vi "ATE_Bandwidth.vi"() -> ()   [LabVIEW 2009]
doc: "Use this template to build a producer/consumer design pattern with events to produce queue items. Use this design pattern instead of the User Interface Event Handler pattern for user interfaces when you want to execute code asynchronously in response to an event without slowing the user interface responsiveness."
uses:
  Rvp8PowerData.ctl
  <vilib>/Analysis/NI_AALPro.lvlib
panel:
  in  "Ready":bool
  out "Instructions":string="rvp8 bandwidth measuring vi\n\nBasic operation:\u0000\u0000\n1 - configure ATE switches with the yellow 'Bandwidth Setup' button\u0000\u0000\n2 - measure the bandwidth with the red 'Calibrate' button\n3 - exit the program with the red 'Exit' button\n\nHints:\nWait for the green 'READY' light before clicking buttons\nClick appropriate blue buttons after making changes on 'Controls' tab\nCheck status tab before calibration"
  out "Real Time XY":cluster{dbl[], dbl[]}(graph)
  in  "Configuration 1":bool
  out "Cal Output File":path
  out "?":cluster{dbl[], dbl[]}[](graph)
  out "RVP8 Bandwidth":cluster{dbl[], dbl[]}[](graph)
  in  "DataSource":bool
  out "File Name":string
  in  "Data Directory":string="/home/operator/ate/data/rvp8_bw"
  in  "Set SigGen":bool
  in  "Initialize":bool
  in  "70 dB":bool
  in  "121 dB":bool
  in  "Switches":bool
  in  "Calibrate":bool
  in  "Stop":bool
  in  "ATE TABS":enum32{"Status", "Controls"}(tab)=enum."Controls"
  out "ATE Switch Status":T1
  out "121dB\nAttenuators":bool[](array[boolean])
  out "70dB\nAttenuators":bool[](array[boolean])
  out "RVP8 Power":T2 {"time" format="%<%H:%M:%S\n%Y/%m/%d>T"}
  out "Signal Generator Status":T3={"Freq (GHz)"=0.0, "RF Power (dBm)"=0.0, "RF Power"=TRUE} {"Freq (GHz)" format="%.5g"; "RF Power (dBm)" format="%.2g"}
  out "121 Verified":bool
  out "70 Verfied":bool
  in  "Center Frequency (GHz)":dbl=2.809 format="%.5g"
  in  "Steps":i32=51
  in  "Steps Size (GHz)":dbl=0.0001 min=0.0 max=0.002 step=1e-06 format="%.5g"
  in  "70 dB Attn":i32=70 min=0 max=70 step=10
  in  "121 dB Attn":i32=121 min=0 max=121 step=1
  in  "ATE Switches":T4
  out "P-State":string
  out "C-State":string
  in  "Busy":bool
  # "RVP8 Bandwidth"
  # "1 dB"
  # "2 dB"
  # "4 dB"
  # "4 dB"
  # "10 dB"
  # "20 dB"
  # "40 dB"
  # "40 dB"
  # "10 dB"
  # "20 dB"
  # "40 dB"
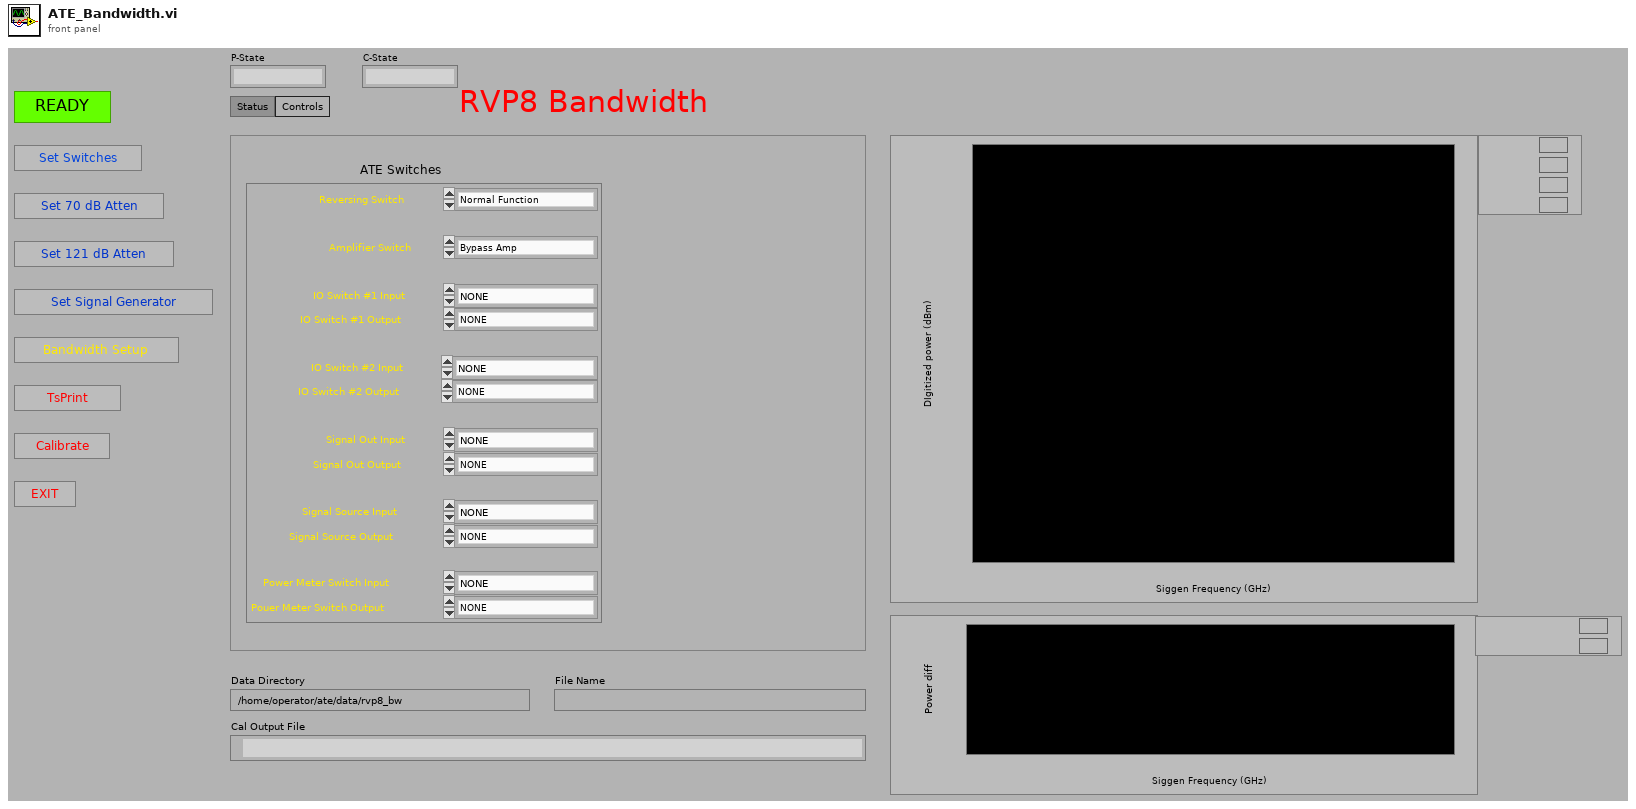
[diagram p1: front panel]
types:
  T1 = cluster{"Reversing Switch ":bool, "IO Switch #1":bool, "IO Switch #2":bool, "Signal Out":bool, "Signal Source":bool, "Power Meter":bool, "Amp By Pass":bool}
  T2 = typedef "Rvp8PowerData.ctl" = cluster{"success":bool, "time":dbl, "el":dbl, "az":dbl, "dbm0":dbl, "dbm1":dbl, "dbmHc":dbl, "dbmHx":dbl, "dbmVc":dbl, "dbmVx":dbl}
  T3 = cluster{"Freq (GHz)":dbl, "RF Power (dBm)":dbl, "RF Power":bool}
  T4 = cluster{"Reversing Switch":enum16{"Normal Function", "Reversing Function"}, "IO Switch #1 Input":enum16{"NONE", "AHR (J2)", "Splitter", "Signal Out Switch (S3)", "Reversing Switch"}, "IO Switch #1 Output":enum16{"NONE", "AHR (J2)", "Delay Device (S4)", "Power Meter Switch (S5)", "Reversing Switch"}, "IO Switch #2 Input":enum16{"NONE", "AVR (J3)", "Splitter", "Signal Out Switch (S3)", " 2W Term (TM1)", "Reversing Switch"}, "IO Switch #2 Output":enum16{"NONE", "AVR (J3)", "Signal Out Switch (S3)", "Power Meter Switch (S5)", "Reversing Switch", "2W Term (TM1)"}, "Signal Out Input":enum16{"NONE", "Amp Bypass Switch (S6)", "IO Switch #1 (S1)", "IO Switch #2 (S2)", "2W Term (TM3)"}, "Signal Out Output":enum16{"NONE", "2 Watt Term (TM3)", "Splitter", "Power Meter Switch (S5)"}, "Signal Source Input":enum16{"NONE", "Delay Device", "Signal Generator (J7)", "Inside Noise Box NF (J5)", "2W Term (TM3)"}, "Signal Source Output":enum16{"NONE", "Amp Bypass Switch", "Test Pulse Generator", "Power Meter Switch (S5)"}, "Power Meter Switch Input":enum16{"NONE", "IO Switch #1 (S1)", "Signal Source Switch (S4)", "Signal Out Switch (S3)", "IO Switch #2 (S2)", "TXH-TXV Switch (J8)"}, "Pouer Meter Switch Output":enum16{"NONE", "Power Meter (J6)"}, "Amplifier Switch":enum16{"Bypass Amp", "Include Amp"}}
  T5 = cluster{"Frequency (GHz)":dbl, "RF Power (dBm)":dbl, "RF ON/OFF":bool}
  T6 = enum16{"open", "replace", "create", "open or create", "replace or create", "replace or create with confirmation"}
  T7 = cluster{"Frequency (GHz)":dbl, "RF Power (dBm)":dbl, "RF Power":bool}
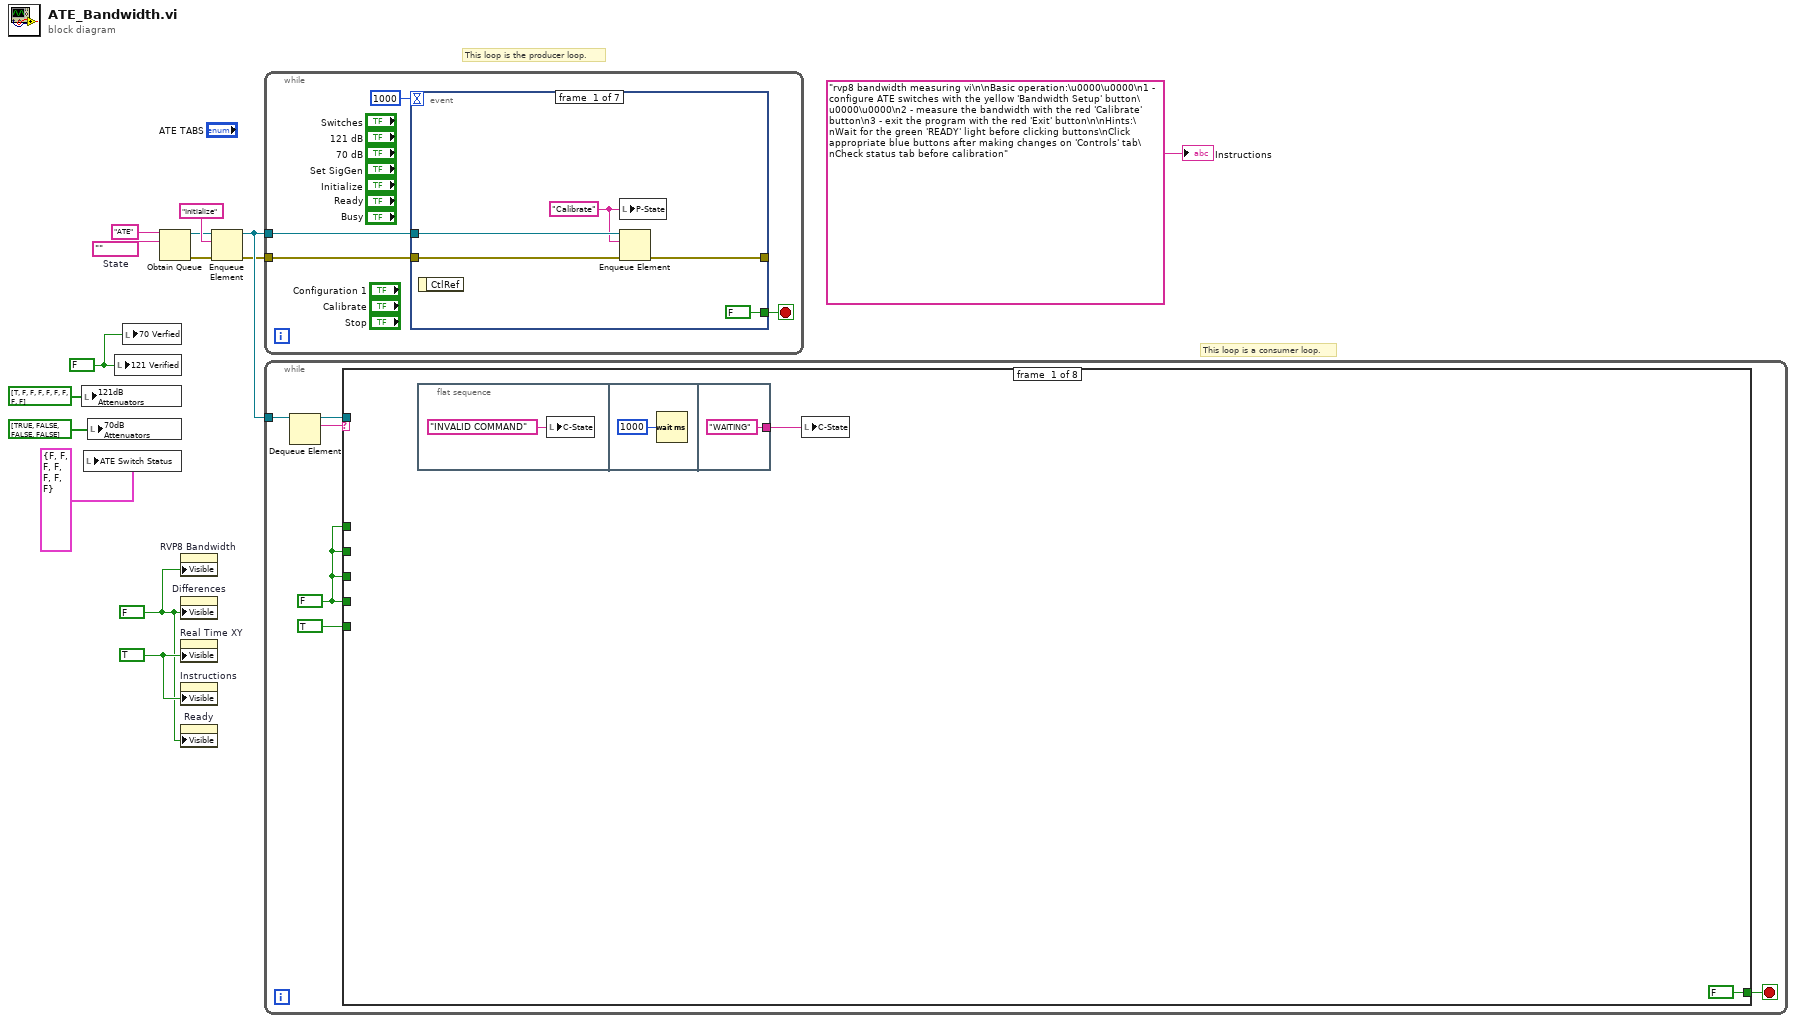
[diagram p0: block diagram]
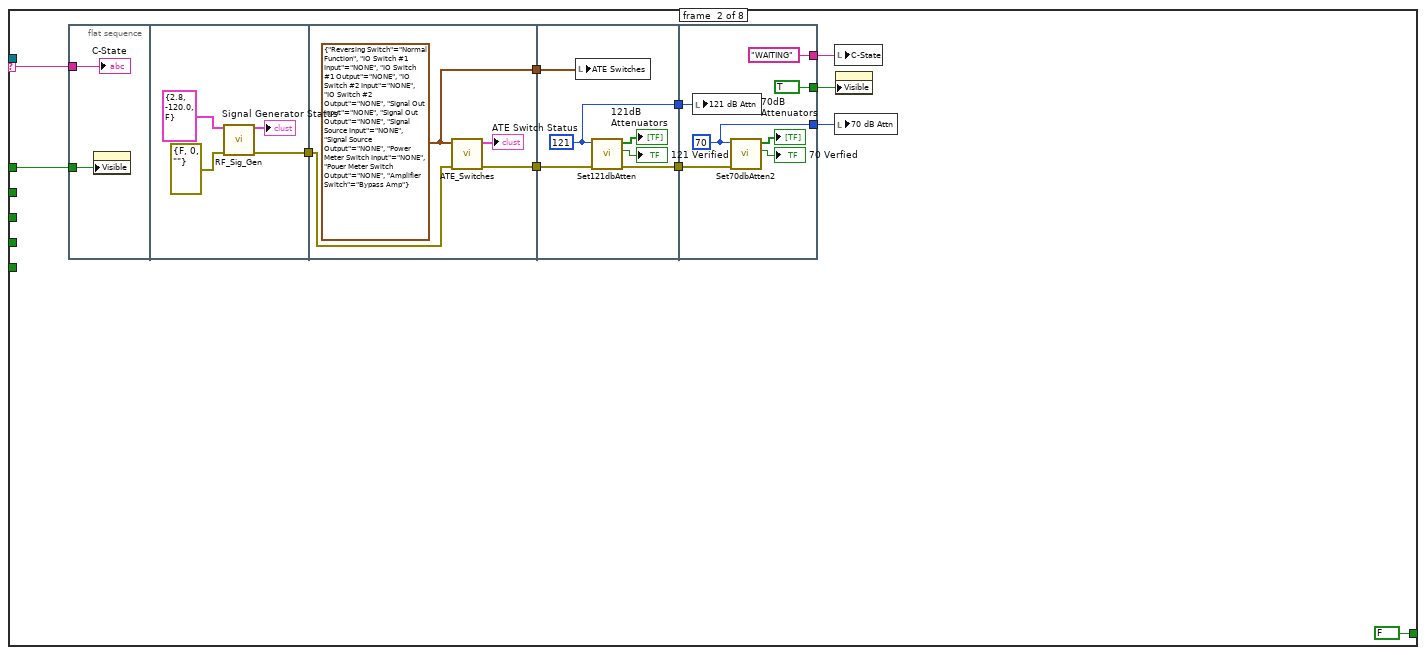
[diagram p2: hidden frame]
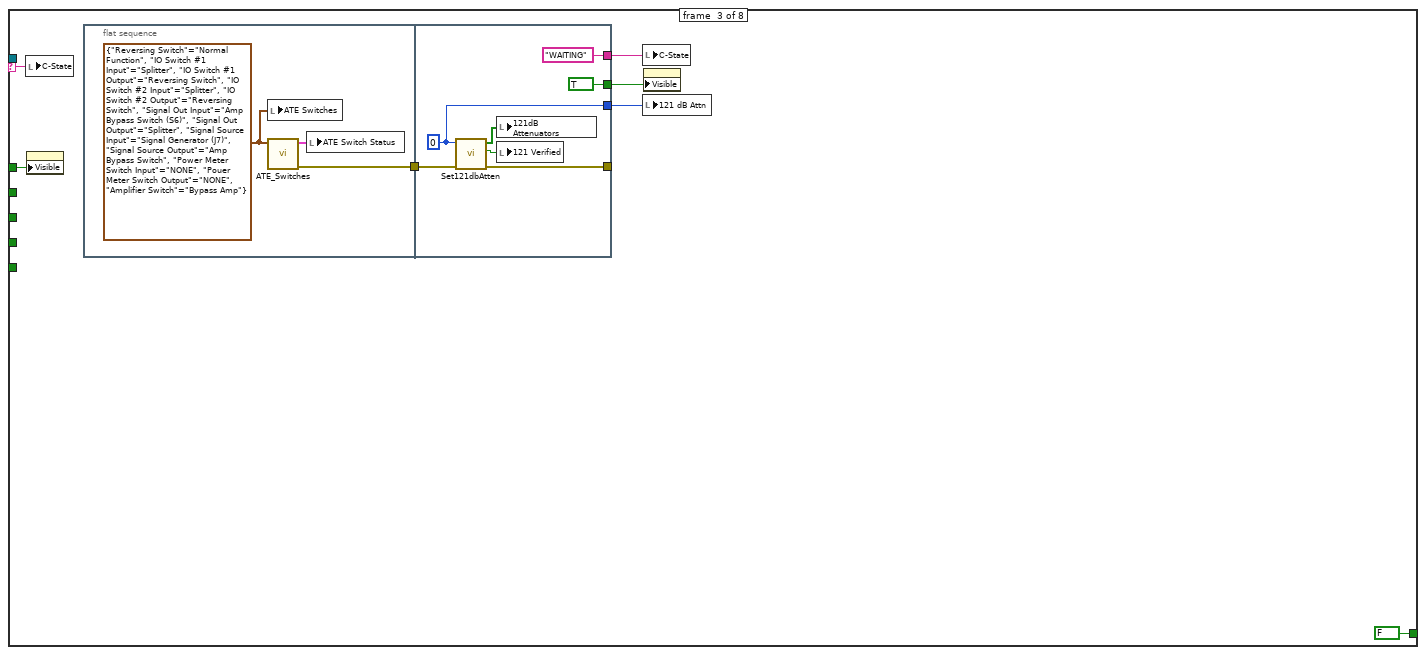
[diagram p3: hidden frame]
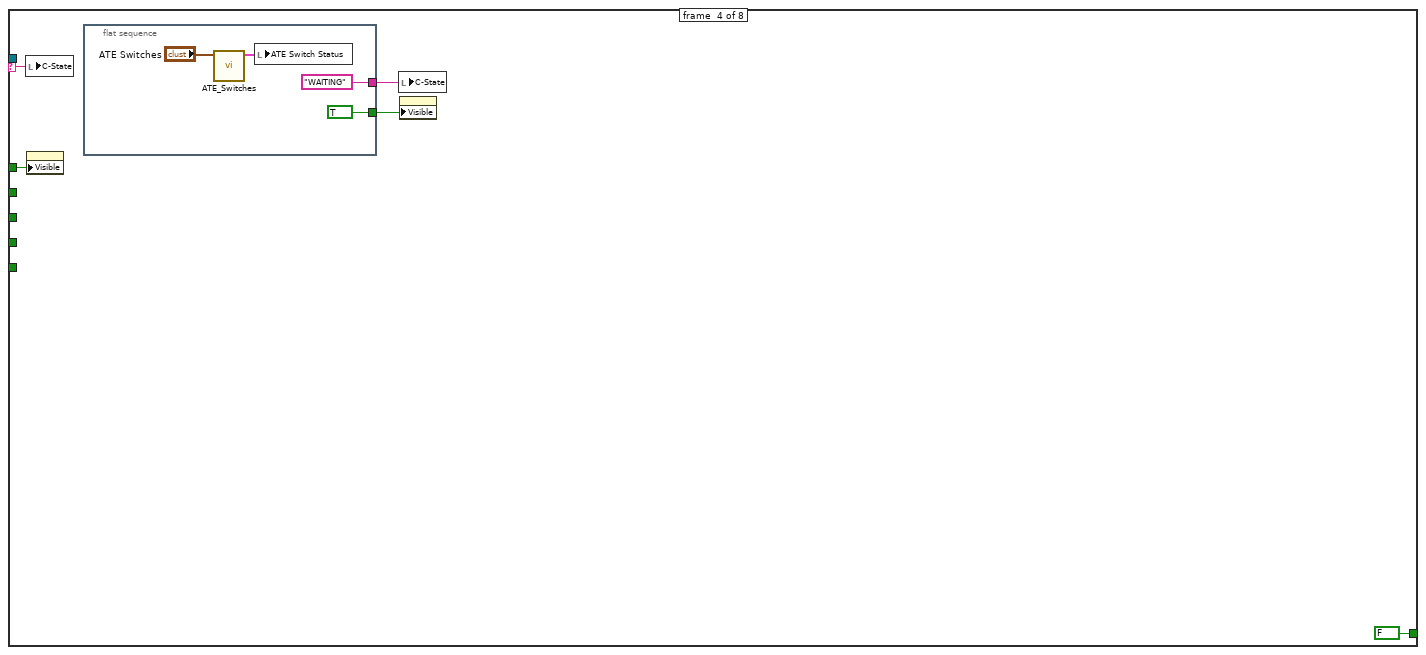
[diagram p4: hidden frame]
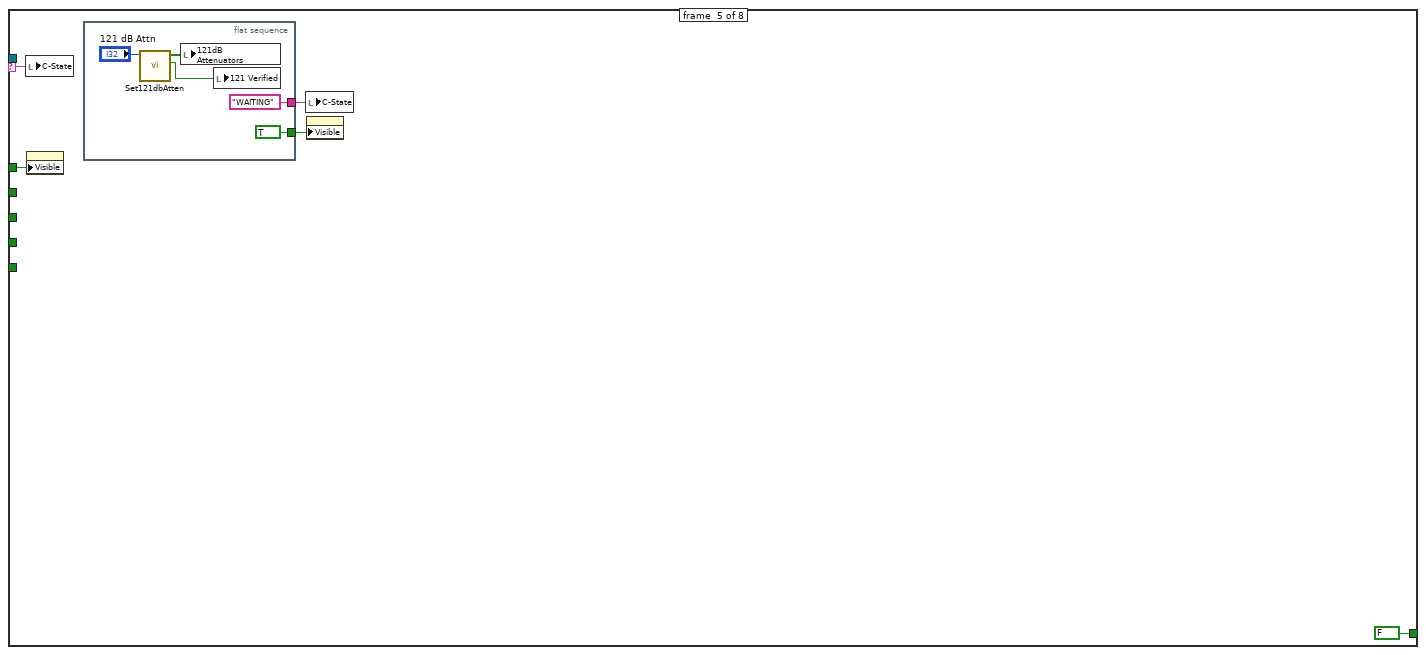
[diagram p5: hidden frame]
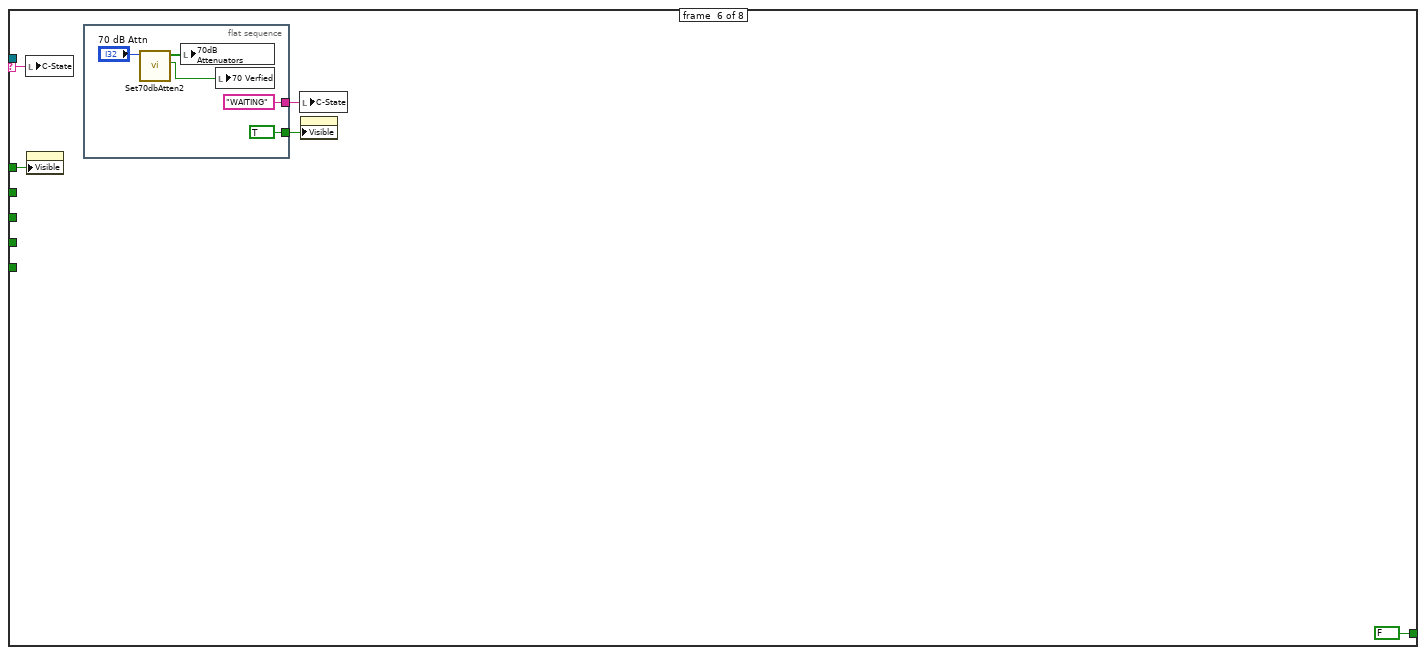
[diagram p6: hidden frame]
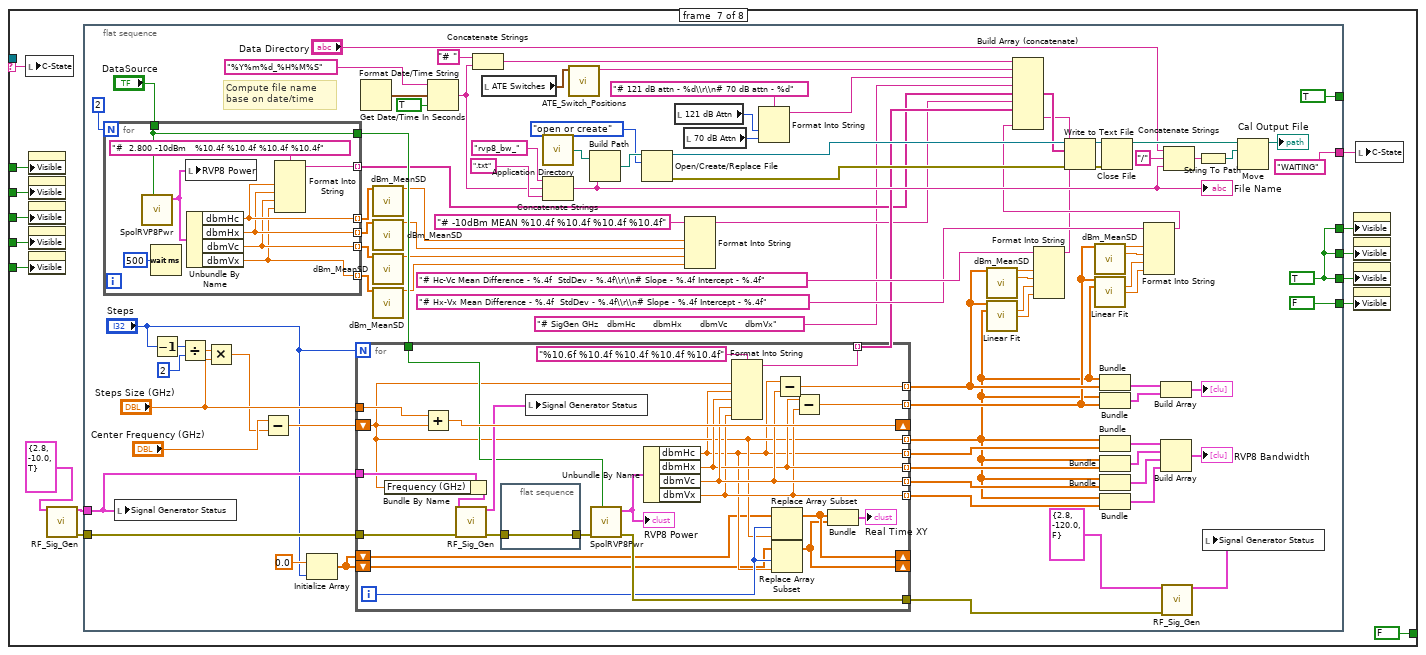
[diagram p7: hidden frame]
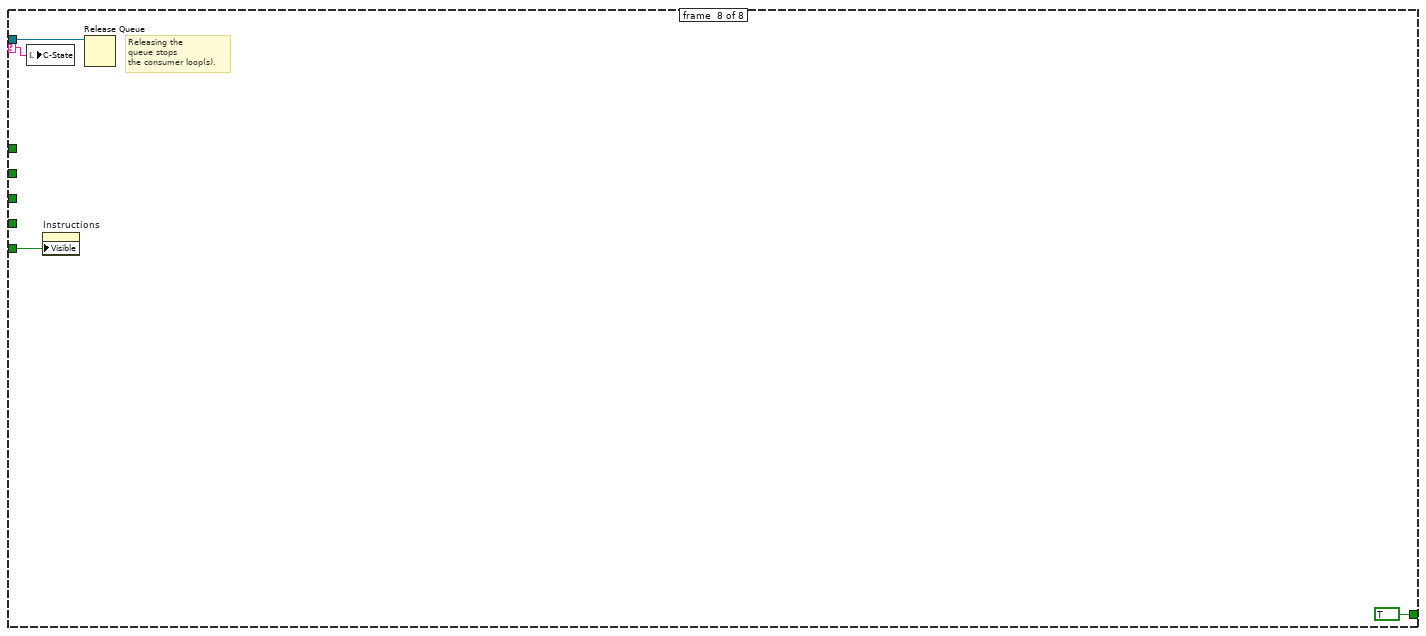
[diagram p8: hidden frame]
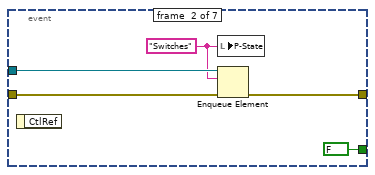
[diagram p9: hidden frame]
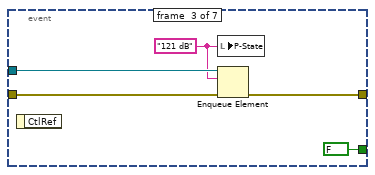
[diagram p10: hidden frame]
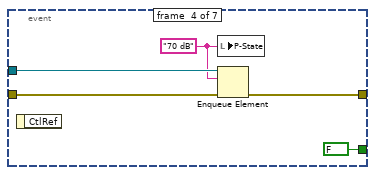
[diagram p11: hidden frame]
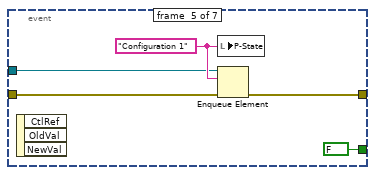
[diagram p12: hidden frame]
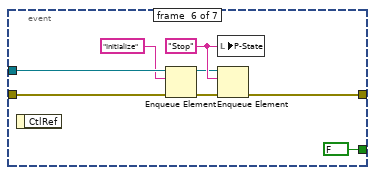
[diagram p13: hidden frame]
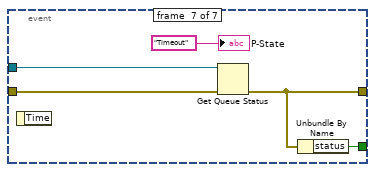
[diagram p14: hidden frame]
diagram:
  w1 = FALSE ("Visible")
  w2 = TRUE ("Visible")
  w4 = FALSE ("70 Verfied")
  w14 = ""  # State
  # "This loop is the producer loop."
  # "This loop is a consumer loop."
  n1 = local write "121dB\nAttenuators"(bool[] [TRUE, FALSE, FALSE, FALSE, FALSE, FALSE, FALSE, FALSE, FALSE] ("121dB\nAttenuators")) -> ()
  n2 = local write "ATE Switch Status"(T1 {"Reversing Switch "=FALSE, "IO Switch #1"=FALSE, "IO Switch #2"=FALSE, "Signal Out"=FALSE, "Signal Source"=FALSE, "Power Meter"=FALSE, "Amp By Pass"=FALSE} ("ATE Switch Status")) -> ()
  n3 = local write "70dB\nAttenuators"(bool[] [TRUE, FALSE, FALSE, FALSE] ("70dB\nAttenuators")) -> ()
  n4 = local write "121 Verified"(w4) -> ()
  n5 = local write "70 Verfied"(w4) -> ()
  n6 = Obtain Queue(name (unnamed)="ATE", element data type=w14) -> (queue out=w11:refnum<queue>, error out=w9:errorcluster)  [unwired: 3 in, 1 out]
  n7 = property on="RVP8 Bandwidth" class="XYGraph (strict)"("Visible"=w1) -> ()  [unwired: 2 in, 2 out]
  n8 = property on="Differences" class="XYGraph (strict)"("Visible"=w1) -> ()  [unwired: 2 in, 2 out]
  n9 = property on="Real Time XY" class="XYGraph (strict)"("Visible"=w2) -> ()  [unwired: 2 in, 2 out]
  n10 = property on="Instructions" class="Str"("Visible"=w2) -> ()  [unwired: 2 in, 2 out]
  n11 = property on="Ready" class="Bool"("Visible"=w1) -> ()  [unwired: 2 in, 2 out]
  n12 = Enqueue Element(queue=w11, element="Initialize", error in (no error)=w9) -> (queue out=w10:refnum<queue>, error out=w8:errorcluster)  [unwired: 1 in, 1 out]
  n13 = while {
    tunnel: w10 -> [w18]
    tunnel: w8 -> [w17]
    stop <- w15 stop-if-true
    n14 = event shown="[6] Timeout" {
      selector: _ -> [_ _ _ _ _ _ _]
      dyn-events: _ -> [_ _ _ _ _ _ _]
      timeout: 1000 -> [_ _ _ _ _ _ _]
      tunnel: w18 -> [w23 w28 w33 w38 w42 w46 w56]
      tunnel: w17 -> [w22 w27 w32 w37 w41 w48 w52]
      tunnel: [w21 w26 w31 w36 w40 w51 w54] -> _
      tunnel: [FALSE FALSE FALSE FALSE FALSE ("status") FALSE w55] -> w15
      event #0 {
        w19 = "Calibrate" ("element")
        n15 = event-data() -> ()  [unwired: 1 in, 1 out]
        n16 = local write "P-State"(w19) -> ()
        n17 = Enqueue Element(queue=w23, element=w19, error in (no error)=w22) -> (error out=w21:errorcluster)  [unwired: 1 in, 2 out]
      }
      event #1 {
        w24 = "Switches" ("element")
        n18 = event-data() -> ()  [unwired: 1 in, 1 out]
        n19 = local write "P-State"(w24) -> ()
        n20 = Enqueue Element(queue=w28, element=w24, error in (no error)=w27) -> (error out=w26:errorcluster)  [unwired: 1 in, 2 out]
      }
      event #2 {
        w29 = "121 dB" ("element")
        n21 = event-data() -> ()  [unwired: 1 in, 1 out]
        n22 = local write "P-State"(w29) -> ()
        n23 = Enqueue Element(queue=w33, element=w29, error in (no error)=w32) -> (error out=w31:errorcluster)  [unwired: 1 in, 2 out]
      }
      event #3 {
        w34 = "70 dB" ("element")
        n24 = event-data() -> ()  [unwired: 1 in, 1 out]
        n25 = local write "P-State"(w34) -> ()
        n26 = Enqueue Element(queue=w38, element=w34, error in (no error)=w37) -> (error out=w36:errorcluster)  [unwired: 1 in, 2 out]
      }
      event #4 {
        w43 = "Configuration 1" ("element")
        n27 = event-data() -> ()  [unwired: 1 in, 3 out]
        n28 = local write "P-State"(w43) -> ()
        n29 = Enqueue Element(queue=w42, element=w43, error in (no error)=w41) -> (error out=w40:errorcluster)  [unwired: 1 in, 2 out]
      }
      event #5 {
        w49 = "Stop" ("element")
        n30 = event-data() -> ()  [unwired: 1 in, 1 out]
        n31 = Enqueue Element(queue=w46, element="Initialize", error in (no error)=w48) -> (queue out=w45:refnum<queue>, error out=w47:errorcluster)  [unwired: 1 in, 1 out]
        n32 = local write "P-State"(w49) -> ()
        n33 = Enqueue Element(queue=w45, element=w49, error in (no error)=w47) -> (error out=w51:errorcluster)  [unwired: 1 in, 2 out]
      }
      event #6 {
        n34 = event-data() -> ()  [unwired: 1 in, 1 out]
        n35 = Get Queue Status(queue=w56, error in (no error)=w52) -> (error out=w54:errorcluster)  [unwired: 1 in, 7 out]
        n36 = Unbundle By Name(w54) -> ("status"=w55:bool)
        "P-State" <- "Timeout" ("element")
      }
    }
  }
  n37 = while {
    tunnel: w10 -> [w62]
    stop <- w59 stop-if-true
    w57 = FALSE ("Visible")
    n38 = Dequeue Element(queue=w62) -> (queue out=w60:refnum<queue>, element=w61:string)  [unwired: 2 in, 2 out]
    n39 = case shown="\"Calibrate\"" w61 {
      selector: w61 -> [_ w68 w104 w123 w131 w141 w161 w292]
      tunnel: w60 -> [_ _ _ _ _ _ _ w291]
      tunnel: [FALSE FALSE FALSE FALSE FALSE FALSE FALSE TRUE] -> w59
      tunnel: w57 -> [_ _ _ _ _ _ w156 _]
      tunnel: w57 -> [_ _ _ _ _ _ w155 _]
      tunnel: TRUE ("Visible") -> [_ _ _ _ _ _ w154 w290]
      tunnel: w57 -> [_ _ _ _ _ _ w150 _]
      tunnel: w57 -> [_ w69 w103 w120 w129 w139 w149 _]
      frame #0 {
        n40 = flat-sequence {
          tunnel: ["WAITING" ("element")] -> w63
          frame #0 {
            n41 = local write "C-State"("INVALID COMMAND" ("C-State")) -> ()
          }
          frame #1 {
            n42 = Wait (ms)(milliseconds to wait=u32 1000) -> ()  [unwired: 1 out]
          }
          frame #2 {
          }
        }
        n43 = local write "C-State"(w63) -> ()
      }
      frame #1 {
        n44 = flat-sequence {
          tunnel: w69 -> [w80]
          tunnel: w68 -> [w79]
          tunnel: [w81] -> w72
          tunnel: [w86] -> w75
          tunnel: w72 -> [w87]
          tunnel: [w85] -> w71
          tunnel: w75 -> [w93]
          tunnel: [w92] -> w76
          tunnel: [w91] -> w74
          tunnel: w71 -> [w89]
          tunnel: ["WAITING" ("element")] -> w77
          tunnel: w76 -> [w100]
          tunnel: w74 -> [w98]
          tunnel: [w97] -> w73
          tunnel: [TRUE ("Visible")] -> w70
          frame #0 {
            n45 = property on="Ready" class="Bool"("Visible"=w80) -> ()  [unwired: 2 in, 2 out]
            "C-State" <- w79
          }
          frame #1 {
            n46 = call "RF_Sig_Gen.vi"("Signal Generator Control"=T5 {"Frequency (GHz)"=2.8, "RF Power (dBm)"=-120.0, "RF ON/OFF"=FALSE}, "error in"=errorcluster {"status"=FALSE, "code"=0, "source"=""}) -> ("Signal Generator Status"=→"Signal Generator Status":T7, "Sig Gen Errors"=w81:errorcluster)  [unwired: 12 in]
          }
          frame #2 {
            w85 = T4 {"Reversing Switch"=enum."Normal Function", "IO Switch #1 Input"=enum."NONE", "IO Switch #1 Output"=enum."NONE", "IO Switch #2 Input"=enum."NONE", "IO Switch #2 Output"=enum."NONE", "Signal Out Input"=enum."NONE", "Signal Out Output"=enum."NONE", "Signal Source Input"=enum."NONE", "Signal Source Output"=enum."NONE", "Power Meter Switch Input"=enum."NONE", "Pouer Meter Switch Output"=enum."NONE", "Amplifier Switch"=enum."Bypass Amp"} ("ATE Switches")
            n47 = call "ATE_Switches.vi"("error in"=w87, "ATE Switches"=w85) -> ("Switch Errors"=w86:errorcluster, "ATE Switch Status"=→"ATE Switch Status":T1)  [unwired: 8 in]
          }
          frame #3 {
            w91 = 121 ("Attenuation (dB)")
            n48 = local write "ATE Switches"(w89) -> ()
            n49 = call "Set121dbAtten.vi"("error in (no error)"=w93, "Attenuation (dB)"=w91) -> ("error out"=w92:errorcluster, "Verfied"=→"121 Verified":bool, "Active Attenuators"=→"121dB\nAttenuators":bool[])  [unwired: 7 in]
          }
          frame #4 {
            w97 = 70 ("Attenuation (dB)")
            n50 = local write "121 dB Attn"(w98) -> ()
            n51 = call "Set70dbAtten2.vi"("error in (no error)"=w100, "Attenuation (dB)"=w97) -> ("Verfied"=→"70 Verfied":bool, "Active Attenuators"=→"70dB\nAttenuators":bool[])  [unwired: 7 in, 1 out]
          }
        }
        n52 = local write "C-State"(w77) -> ()
        n53 = local write "70 dB Attn"(w73) -> ()
        n54 = property on="Ready" class="Bool"("Visible"=w70) -> ()  [unwired: 2 in, 2 out]
      }
      frame #2 {
        n55 = local write "C-State"(w104) -> ()
        n56 = property on="Ready" class="Bool"("Visible"=w103) -> ()  [unwired: 2 in, 2 out]
        n57 = flat-sequence {
          tunnel: [w111] -> w107
          tunnel: w107 -> [w118]
          tunnel: [w113] -> w106
          tunnel: ["WAITING" ("element")] -> w105
          tunnel: [w116] -> _
          tunnel: [TRUE ("Visible")] -> w102
          frame #0 {
            w109 = T4 {"Reversing Switch"=enum."Normal Function", "IO Switch #1 Input"=enum."Splitter", "IO Switch #1 Output"=enum."Reversing Switch", "IO Switch #2 Input"=enum."Splitter", "IO Switch #2 Output"=enum."Reversing Switch", "Signal Out Input"=enum."Amp Bypass Switch (S6)", "Signal Out Output"=enum."Splitter", "Signal Source Input"=enum."Signal Generator (J7)", "Signal Source Output"=enum."Amp Bypass Switch", "Power Meter Switch Input"=enum."NONE", "Pouer Meter Switch Output"=enum."NONE", "Amplifier Switch"=enum."Bypass Amp"} ("ATE Switches")
            n58 = local write "ATE Switches"(w109) -> ()
            n59 = call "ATE_Switches.vi"("ATE Switches"=w109) -> ("Switch Errors"=w111:errorcluster, "ATE Switch Status"=w110:T1)  [unwired: 9 in]
            n60 = local write "ATE Switch Status"(w110) -> ()
          }
          frame #1 {
            w113 = 0 ("Attenuation (dB)")
            n61 = call "Set121dbAtten.vi"("error in (no error)"=w118, "Attenuation (dB)"=w113) -> ("error out"=w116:errorcluster, "Verfied"=w114:bool, "Active Attenuators"=w115:bool[])  [unwired: 7 in]
            n62 = local write "121dB\nAttenuators"(w115) -> ()
            n63 = local write "121 Verified"(w114) -> ()
          }
        }
        n64 = local write "C-State"(w105) -> ()
        n65 = local write "121 dB Attn"(w106) -> ()
        n66 = property on="Ready" class="Bool"("Visible"=w102) -> ()  [unwired: 2 in, 2 out]
      }
      frame #3 {
        n67 = local write "C-State"(w123) -> ()
        n68 = property on="Ready" class="Bool"("Visible"=w120) -> ()  [unwired: 2 in, 2 out]
        n69 = flat-sequence {
          tunnel: ["WAITING" ("element")] -> w121
          tunnel: [TRUE ("Visible")] -> w119
          frame #0 {
            n70 = call "ATE_Switches.vi"("ATE Switches"="ATE Switches") -> ("ATE Switch Status"=w126:T1)  [unwired: 9 in, 1 out]
            n71 = local write "ATE Switch Status"(w126) -> ()
          }
        }
        n72 = local write "C-State"(w121) -> ()
        n73 = property on="Ready" class="Bool"("Visible"=w119) -> ()  [unwired: 2 in, 2 out]
      }
      frame #4 {
        n74 = local write "C-State"(w131) -> ()
        n75 = property on="Ready" class="Bool"("Visible"=w129) -> ()  [unwired: 2 in, 2 out]
        n76 = flat-sequence {
          tunnel: ["WAITING" ("element")] -> w130
          tunnel: [TRUE ("Visible")] -> w128
          frame #0 {
            n77 = call "Set121dbAtten.vi"("Attenuation (dB)"="121 dB Attn") -> ("Verfied"=w135:bool, "Active Attenuators"=w137:bool[])  [unwired: 8 in, 1 out]
            n78 = local write "121dB\nAttenuators"(w137) -> ()
            n79 = local write "121 Verified"(w135) -> ()
          }
        }
        n80 = local write "C-State"(w130) -> ()
        n81 = property on="Ready" class="Bool"("Visible"=w128) -> ()  [unwired: 2 in, 2 out]
      }
      frame #5 {
        n82 = local write "C-State"(w141) -> ()
        n83 = property on="Ready" class="Bool"("Visible"=w139) -> ()  [unwired: 2 in, 2 out]
        n84 = flat-sequence {
          tunnel: ["WAITING" ("element")] -> w140
          tunnel: [TRUE ("Visible")] -> w138
          frame #0 {
            n85 = call "Set70dbAtten2.vi"("Attenuation (dB)"="70 dB Attn") -> ("Verfied"=w144:bool, "Active Attenuators"=w146:bool[])  [unwired: 8 in, 1 out]
            n86 = local write "70dB\nAttenuators"(w146) -> ()
            n87 = local write "70 Verfied"(w144) -> ()
          }
        }
        n88 = local write "C-State"(w140) -> ()
        n89 = property on="Ready" class="Bool"("Visible"=w138) -> ()  [unwired: 2 in, 2 out]
      }
      frame #6 {
        n90 = local write "C-State"(w161) -> ()
        n91 = property on="Ready" class="Bool"("Visible"=w149) -> ()  [unwired: 2 in, 2 out]
        n92 = property on="Instructions" class="Str"("Visible"=w150) -> ()  [unwired: 2 in, 2 out]
        n93 = property on="RVP8 Bandwidth" class="XYGraph (strict)"("Visible"=w156) -> ()  [unwired: 2 in, 2 out]
        n94 = property class="XYGraph (strict)"("Visible"=w155) -> ()  [unwired: 2 in, 2 out]
        n95 = property on="Real Time XY" class="XYGraph (strict)"("Visible"=w154) -> ()  [unwired: 2 in, 2 out]
        n96 = call "RF_Sig_Gen.vi"("Signal Generator Control"=T5 {"Frequency (GHz)"=2.8, "RF Power (dBm)"=-10.0, "RF ON/OFF"=TRUE}) -> ("Signal Generator Status"=w159:T7, "Sig Gen Errors"=w158:errorcluster)  [unwired: 13 in]
        n97 = flat-sequence {
          tunnel: ["WAITING" ("element")] -> w160
          tunnel: w159 -> [w176]
          tunnel: w158 -> [w177]
          tunnel: [w165] -> w153
          tunnel: [w165] -> w152
          tunnel: [FALSE ("Visible")] -> w151
          tunnel: [TRUE ("Visible")] -> _
          tunnel: [w165] -> w148
          frame #0 {
            w165 = TRUE ("Visible")
            # "Compute file name base on date/time"
            n98 = for {
              N: 2 -> [_]
              tunnel: [w260] -> w181 mode=indexing
              tunnel: [w259] -> w194 mode=indexing
              tunnel: [w258] -> w195 mode=indexing
              tunnel: [w257] -> w196 mode=indexing
              tunnel: [w254] -> w197 mode=indexing
              tunnel: "DataSource" -> [w256]
              tunnel: [w256] -> w191
              n99 = call "SpolRVP8Pwr.vi"("DataSource"=w256) -> ("RVP8_power"=w255:T2)  [unwired: 7 in, 3 out]
              n100 = Wait (ms)(milliseconds to wait=u32 500) -> ()  [unwired: 1 out]
              n101 = local write "RVP8 Power"(w255) -> ()
              n102 = Unbundle By Name(w255) -> ("dbmHc"=w259:dbl, "dbmHx"=w258:dbl, "dbmVc"=w257:dbl, "dbmVx"=w254:dbl)
              n103 = Format Into String(format string="#  2.800 -10dBm   %10.4f %10.4f %10.4f %10.4f", w259, w258, w257, w254) -> (resulting string=w260:string)  [unwired: 2 in, 1 out]
            }
            n104 = local write "Signal Generator Status"(w176) -> ()
            n105 = Decrement(x="Steps") -> (x-1=w179:i32)
            n106 = Divide(x=w179, y=2) -> (x/y=w175:dbl)
            n107 = Multiply(x=w175, y="Steps Size (GHz)") -> (x*y=w171:dbl)
            n108 = Subtract(x="Center Frequency (GHz)", y=w171) -> (x-y=w174:dbl)
            n109 = Initialize Array(0.0 ("element"), "Steps") -> (w168:dbl[])
            n110 = for {
              N: "Steps" -> [_]
              shift-right: [w277] -> _
              shift-left: w174 -> [w268]
              tunnel: w177 -> [w285]
              tunnel: [w268] -> w211 mode=indexing
              tunnel: [w267] -> w246 mode=indexing
              tunnel: [w275] -> w245 mode=indexing
              tunnel: [w276] -> w244 mode=indexing
              tunnel: [w274] -> w243 mode=indexing
              tunnel: [w288] -> w183 mode=indexing
              tunnel: [w279] -> w213 mode=indexing
              tunnel: [w278] -> w212 mode=indexing
              tunnel: w176 -> [w286]
              tunnel: [w282] -> w223
              tunnel: w191 -> [w272]
              tunnel: "Steps Size (GHz)" -> [w271]
              shift-right: [w264] -> _
              shift-left: w168 -> [w265]
              shift-right: [w263] -> _
              shift-left: w168 -> [w266]
              i -> [w269]
              n111 = Bundle By Name(cluster=w286, "Frequency (GHz)"=w268) -> (w280:T7)
              n112 = Add(x=w271, y=w268) -> (x+y=w277:dbl)
              n113 = call "RF_Sig_Gen.vi"("Signal Generator Control"=w280, "error in"=w285) -> ("Signal Generator Status"=w273:T7, "Sig Gen Errors"=w284:errorcluster)  [unwired: 12 in]
              n114 = flat-sequence {
                tunnel: w284 -> [w289]
                tunnel: [w289] -> w283
                frame #0 {
                }
              }
              n115 = local write "Signal Generator Status"(w273) -> ()
              n116 = call "SpolRVP8Pwr.vi"("DataSource"=w272, "error in (no error)"=w283) -> ("Comm error"=w282:errorcluster, "RVP8_power"=w287:T2)  [unwired: 6 in, 2 out]
              "RVP8 Power" <- w287
              n117 = Unbundle By Name(w287) -> ("dbmHc"=w267:dbl, "dbmHx"=w275:dbl, "dbmVc"=w276:dbl, "dbmVx"=w274:dbl)
              n118 = Format Into String(format string="%10.6f %10.4f %10.4f %10.4f %10.4f", w268, w267, w275, w276, w274) -> (resulting string=w288:string)  [unwired: 2 in, 1 out]
              n119 = Replace Array Subset(array=w265, new element=w268, index=w269) -> (w264:dbl[])
              n120 = Replace Array Subset(array=w266, new element=w267, index=w269) -> (w263:dbl[])
              n121 = Subtract(x=w267, y=w276) -> (x-y=w279:dbl)
              n122 = Subtract(x=w275, y=w274) -> (x-y=w278:dbl)
              n123 = Bundle(w264, w263) -> (→"Real Time XY":cluster{dbl[], dbl[]})  [unwired: 1 in]
            }
            n124 = Get Date/Time In Seconds() -> (seconds since 1Jan1904=w248:timestamp)
            n125 = call "dBm_MeanSD.vi"("dBm array"=w194) -> ("dBm mean"=w188:dbl)  [unwired: 13 in, 1 out]
            n126 = call "dBm_MeanSD.vi"("dBm array"=w195) -> ("dBm mean"=w187:dbl)  [unwired: 13 in, 1 out]
            n127 = call "dBm_MeanSD.vi"("dBm array"=w196) -> ("dBm mean"=w186:dbl)  [unwired: 13 in, 1 out]
            n128 = call "dBm_MeanSD.vi"("dBm array"=w197) -> ("dBm mean"=w189:dbl)  [unwired: 13 in, 1 out]
            n129 = Format Date/Time String(time format string (%c)="%Y%m%d_%H%M%S", seconds (now)=w248, UTC format=TRUE) -> (date/time string=w204:string)
            n130 = Concatenate Strings("# " ("string"), w204) -> (w203:string)
            n131 = local read "ATE Switches"() -> (w221:T4)
            n132 = call <vilib>:"Application Directory.vi"() -> ("Application Directory"=w247:path)
            n133 = Concatenate Strings("rvp8_bw_", w204, ".txt") -> (w200:string)
            "File Name" <- w200
            n134 = call "ATE_Switch_Positions.vi"("ATE Switches"=w221) -> ("ATE Switch/Position"=w202:string)  [unwired: 10 in]
            n135 = Build Path(base path=w247, name or relative path=w200) -> (appended path=w234:path)
            n136 = Open/Create/Replace File(file path (use dialog)=w234, operation (0:open)=T6."open or create") -> (refnum out=w233:refnum<file>, error out=w232:errorcluster)  [unwired: 4 in, 1 out]
            n137 = local read "121 dB Attn"() -> (w218:i32)
            n138 = local read "70 dB Attn"() -> (w217:i32)
            n139 = Format Into String(format string="# -10dBm MEAN %10.4f %10.4f %10.4f %10.4f", w188, w187, w186, w189) -> (resulting string=w182:string)  [unwired: 2 in, 1 out]
            n140 = Format Into String(format string="# 121 dB attn - %d\\r\\n# 70 dB attn - %d", w218, w217) -> (resulting string=w201:string)  [unwired: 2 in, 1 out]
            n141 = call "dBm_MeanSD.vi"("dBm array"=w213) -> ("dBm mean"=w216:dbl, "Std Dev"=w163:dbl)  [unwired: 13 in]
            n142 = call <vilib>:"Linear Fit.vi"("Y"=w213, "X"=w211) -> ("slope"=w215:dbl, "intercept"=w214:dbl)  [unwired: 9 in, 3 out]
            n143 = Format Into String(format string="# Hc-Vc Mean Difference - %.4f  StdDev - %.4f\\r\\n# Slope - %.4f Intercept - %.4f", w216, w163, w215, w214) -> (resulting string=w184:string)  [unwired: 2 in, 1 out]
            n144 = call "dBm_MeanSD.vi"("dBm array"=w212) -> ("dBm mean"=w210:dbl, "Std Dev"=w164:dbl)  [unwired: 13 in]
            n145 = call <vilib>:"Linear Fit.vi"("Y"=w212, "X"=w211) -> ("slope"=w209:dbl, "intercept"=w208:dbl)  [unwired: 9 in, 3 out]
            n146 = Bundle(w211, w213) -> (w242:cluster{dbl[], dbl[]})  [unwired: 1 in]
            n147 = Bundle(w211, w212) -> (w241:cluster{dbl[], dbl[]})  [unwired: 1 in]
            n148 = Bundle(w211, w246) -> (w240:cluster{dbl[], dbl[]})  [unwired: 1 in]
            n149 = Bundle(w211, w245) -> (w239:cluster{dbl[], dbl[]})  [unwired: 1 in]
            n150 = Bundle(w211, w244) -> (w237:cluster{dbl[], dbl[]})  [unwired: 1 in]
            n151 = Bundle(w211, w243) -> (w238:cluster{dbl[], dbl[]})  [unwired: 1 in]
            n152 = Format Into String(format string="# Hx-Vx Mean Difference - %.4f  StdDev - %.4f\\r\\n# Slope - %.4f Intercept - %.4f", w210, w164, w209, w208) -> (resulting string=w185:string)  [unwired: 2 in, 1 out]
            n153 = Build Array (concatenate)(w203, w202, w201, "# SigGen GHz   dbmHc      dbmHx      dbmVc      dbmVx", w181, w182, w183, w184, w185) -> (w220:string[])
            n154 = Write to Text File(file (use dialog)=w233, text=w220, error in=w232) -> (refnum out=w231:refnum<file>, error out=w230:errorcluster)  [unwired: 1 in, 1 out]
            n155 = Close File(refnum=w231, error in=w230) -> (path=w227:path)  [unwired: 1 out]
            n156 = Build Array(w242, w241) -> (→"?":cluster{dbl[], dbl[]}[])
            n157 = Build Array(w240, w239, w237, w238) -> (→"RVP8 Bandwidth":cluster{dbl[], dbl[]}[])
            n158 = call "RF_Sig_Gen.vi"("Signal Generator Control"=T5 {"Frequency (GHz)"=2.8, "RF Power (dBm)"=-120.0, "RF ON/OFF"=FALSE}, "error in"=w223) -> ("Signal Generator Status"=w224:T7)  [unwired: 12 in, 1 out]
            n159 = Concatenate Strings("Data Directory", "/" ("string"), w200) -> (w228:string)
            n160 = String To Path(string=w228) -> (path=w226:path)
            n161 = local write "Signal Generator Status"(w224) -> ()
            n162 = Move(source path=w227, 10:w226) -> (3:→"Cal Output File":path)  [unwired: 3 in, 2 out]
          }
        }
        n163 = property on="Ready" class="Bool"("Visible"=w148) -> ()  [unwired: 2 in, 2 out]
        n164 = property on="RVP8 Bandwidth" class="XYGraph (strict)"("Visible"=w153) -> ()  [unwired: 2 in, 2 out]
        n165 = property class="XYGraph (strict)"("Visible"=w152) -> ()  [unwired: 2 in, 2 out]
        n166 = property on="Real Time XY" class="XYGraph (strict)"("Visible"=w151) -> ()  [unwired: 2 in, 2 out]
        n167 = local write "C-State"(w160) -> ()
      }
      frame #7 {
        # "Releasing the\nqueue stops\nthe consumer loop(s)."
        n168 = local write "C-State"(w292) -> ()
        n169 = property on="Instructions" class="Str"("Visible"=w290) -> ()  [unwired: 2 in, 2 out]
        n170 = Release Queue(queue=w291) -> ()  [unwired: 2 in, 3 out]
      }
    }
  }
  "Instructions" <- "rvp8 bandwidth measuring vi\n\nBasic operation:\u0000\u0000\n1 - configure ATE switches with the yellow 'Bandwidth Setup' button\u0000\u0000\n2 - measure the bandwidth with the red 'Calibrate' button\n3 - exit the program with the red 'Exit' button\n\nHints:\nWait for the green 'READY' light before clicking buttons\nClick appropriate blue buttons after making changes on 'Controls' tab\nCheck status tab before calibration" ("String")
